vi "collision_avoid.vi"(7 "x0":dbl format="%#_13g", 8 "d":dbl=3.0 format="%#_13g", 9 "x3":dbl=25.0 format="%#_13g", 10 "x2":dbl=11.0 format="%#_13g", 11 "x1":dbl=7.0 format="%#_13g") -> (0 "y":dbl[](array[numeric]), 3 "x":dbl[](array[numeric]))   [LabVIEW 2015]
panel:
  out "XY Graph":cluster{"Y":dbl[], "Y":dbl[]}[](graph)
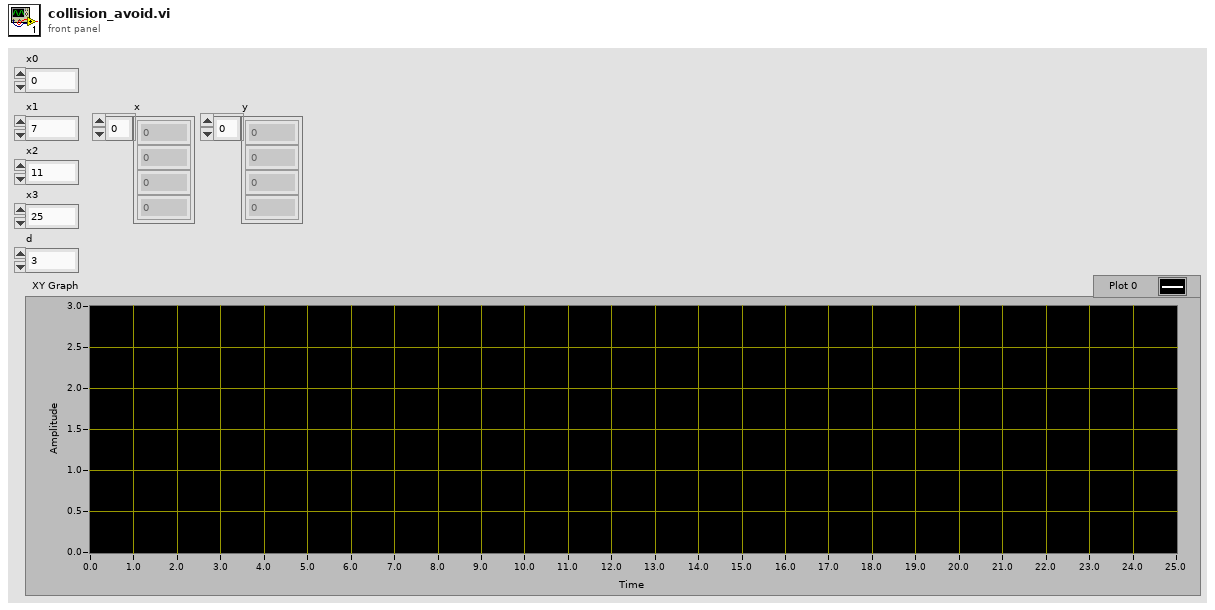
[diagram p1: front panel]
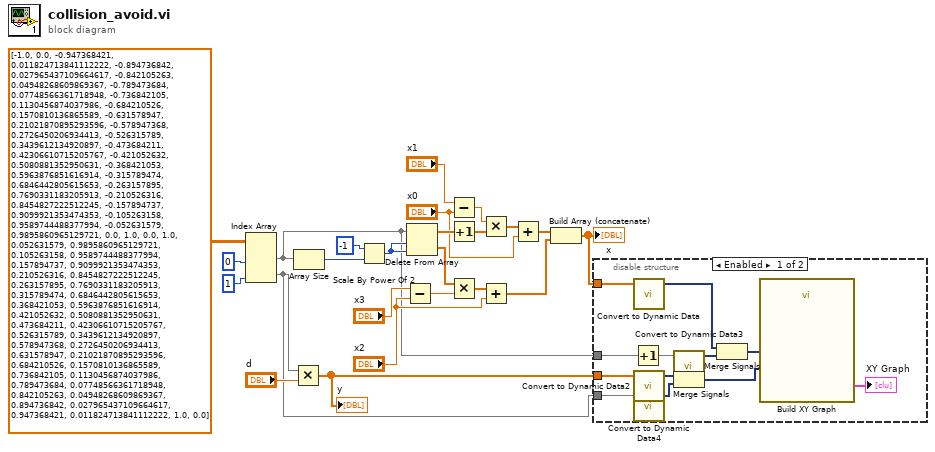
[diagram p0: block diagram]
diagram:
  n1 = Index Array(array=dbl[][] [[-1.0, 0.0], [-0.947368421, 0.011824713841112222], [-0.894736842, 0.027965437109664617], [-0.842105263, 0.04948268609869367], [-0.789473684, 0.07748566361718948], [-0.736842105, 0.1130456874037986], [-0.684210526, 0.1570810136865589], [-0.631578947, 0.21021870895293596], [-0.578947368, 0.2726450206934413], [-0.526315789, 0.3439612134920897], [-0.473684211, 0.42306610715205767], [-0.421052632, 0.5080881352950631], [-0.368421053, 0.5963876851616914], [-0.315789474, 0.6846442805615653], [-0.263157895, 0.7690331183205913], [-0.210526316, 0.8454827222512245], [-0.157894737, 0.9099921353474353], [-0.105263158, 0.9589744488377994], [-0.052631579, 0.9895860965129721], [0.0, 1.0], [0.0, 1.0], [0.052631579, 0.9895860965129721], [0.105263158, 0.9589744488377994], [0.157894737, 0.9099921353474353], [0.210526316, 0.8454827222512245], [0.263157895, 0.7690331183205913], [0.315789474, 0.6846442805615653], [0.368421053, 0.5963876851616914], [0.421052632, 0.5080881352950631], [0.473684211, 0.42306610715205767], [0.526315789, 0.3439612134920897], [0.578947368, 0.2726450206934413], [0.631578947, 0.21021870895293596], [0.684210526, 0.1570810136865589], [0.736842105, 0.1130456874037986], [0.789473684, 0.07748566361718948], [0.842105263, 0.04948268609869367], [0.894736842, 0.027965437109664617], [0.947368421, 0.011824713841112222], [1.0, 0.0]] ("appended array"), index (col) #1=0 ("disabled index (col)"), index (col) #2=1 ("index (col)")) -> (element #1=w7:dbl[], element #2=w6:dbl[])  [unwired: 2 in]
  n2 = Multiply(x=w6, y="d") -> (x*y=w15:dbl[])
  "y" <- w15
  n3 = Array Size(array=w7) -> (size(s)=w14:i32)
  n4 = Scale By Power Of 2(n=i16 -1, x=w14) -> (x*2^n=w10:i32)
  n5 = Subtract(x="x3", y="x2") -> (x-y=w22:dbl)
  n6 = Delete From Array(array=w7, length=w10, index=w10) -> (deleted portion=w12:dbl[], array with subset deleted=w11:dbl[])
  n7 = Subtract(x="x1", y="x0") -> (x-y=w4:dbl)
  n8 = Increment(x=w11) -> (x+1=w9:dbl[])
  n9 = Multiply(x=w12, y=w22) -> (x*y=w21:dbl[])
  n10 = Multiply(x=w4, y=w9) -> (x*y=w3:dbl[])
  n11 = Add(x=w21, y="x2") -> (x+y=w17:dbl[])
  n12 = Add(x=w3, y="x0") -> (x+y=w1:dbl[])
  n13 = Build Array (concatenate)(w1, w17) -> (w16:dbl[])
  "x" <- w16
  n14 = disable-structure shown="Enabled" {
    disable-tunnel: w16 -> [w35 _]
    disable-tunnel: w15 -> [w33 _]
    disable-tunnel: w7 -> [w26 _]
    disable-tunnel: w6 -> [w28 _]
    frame Enabled {
      n15 = Increment(x=w26) -> (x+1=w25:dbl[])
      n16 = call "Convert to Dynamic Data"("Array"=w35) -> ("Dynamic Data Type"=w34:dynamicdata)  [unwired: 3 in]
      n17 = call "Convert to Dynamic Data2"("Array"=w33) -> ("Dynamic Data Type"=w32:dynamicdata)  [unwired: 3 in]
      n18 = call "Convert to Dynamic Data4"("Array"=w28) -> ("Dynamic Data Type"=w27:dynamicdata)  [unwired: 3 in]
      n19 = call "Convert to Dynamic Data3"("Array"=w25) -> ("Dynamic Data Type"=w30:dynamicdata)  [unwired: 3 in]
      n20 = Merge Signals(w32, w27) -> (w29:dynamicdata)
      n21 = Merge Signals(w34, w30) -> (w31:dynamicdata)
      n22 = call "Build XY Graph"("Y Input"=w29, "X Input"=w31) -> ("XY Graph"=→"XY Graph":cluster{"X":dbl[], "Y":dbl[]}[])  [unwired: 8 in, 1 out]
    }
    frame Disabled {
    }
  }
